vi "Polynomial Eigenvalue Problem (DBL, Spec Case).vi"(10 "output option":i32(ring)=1 items=["eigenvalues", "eigenvalues & vectors"], 11 "Input Matrices":dbl[][][](array[numeric])) -> (0 "error":i32, 2 "Eigenvectors":T1, 3 "Eigenvalues":cdb[](array[numeric]))   [LabVIEW 2020, in "NI_AALPro.lvlib"]
uses:
  <vilib>/Analysis/NI_AALPro.lvlib
  <vilib>/Analysis/Matrix/Datatypes/ComplexMatrix.ctl
  <vilib>/Analysis/7linalg.llb/Real Generalized Eigenvalues and Vectors.vi
  <vilib>/Analysis/7linalg.llb/Real Eigenvalues and Vectors.vi
  <vilib>/Analysis/Matrix/NI_Matrix.lvlib
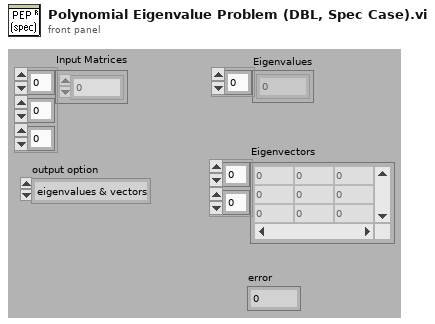
[diagram p1: front panel]
types:
  T1 = typedef "NI_Matrix.lvlib/ComplexMatrix.ctl" = cdb[][]
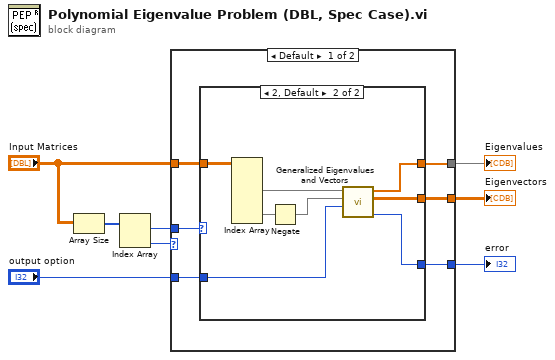
[diagram p0: block diagram]
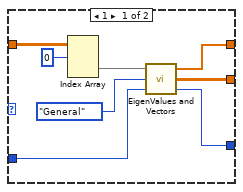
[diagram p2: hidden frame]
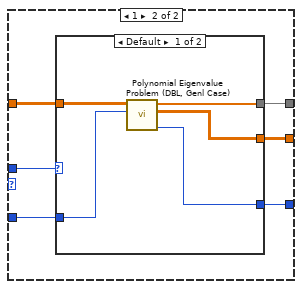
[diagram p3: hidden frame]
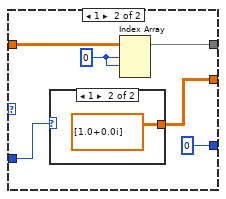
[diagram p4: hidden frame]
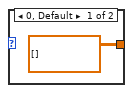
[diagram p5: hidden frame]
diagram:
  n1 = Array Size(array="Input Matrices") -> (size(s)=w8:i32[])
  n2 = Index Array(array=w8) -> (element #1=w6:i32, element #2=w7:i32)  [unwired: 2 in]
  n3 = case shown="Default" w7 {
    tunnel: w6 -> [w14 w36]
    tunnel: "Input Matrices" -> [w13 w35]
    tunnel: [w12 w34] -> w4
    tunnel: [w11 w33] -> w3
    tunnel: [w10 w32] -> w2
    tunnel: "output option" -> [w9 w31]
    frame Default {
      n4 = case shown="2, Default" w14 {
        tunnel: w13 -> [w22 w30]
        tunnel: [w18 w26] -> w12
        tunnel: [w17 w25] -> w11
        tunnel: [w16 w24] -> w10
        tunnel: w9 -> [w15 w23]
        frame 1 {
          n5 = Index Array(array=w22, index (dim 0)=0 ("index (page)")) -> (element=w20:dbl[][])  [unwired: 2 in]
          n6 = call-poly <vilib>:"EigenValues and Vectors.vi"("output option"=w15, "matrix type"=enum32{"General", "Symmetric"}."General", "Input Matrix"=w20) -> ("error"=w16:i32, "Eigenvectors"=w17:T1, "Eigenvalues"=w18:cdb[])
        }
        frame 2, Default {
          n7 = Index Array(array=w30) -> (element #1=w28:dbl[][], element #2=w29:dbl[][])  [unwired: 6 in]
          n8 = Negate(x=w29) -> (-x=w27:dbl[][])
          n9 = call-poly <vilib>:"Generalized Eigenvalues and Vectors.vi"("output option"=w23, "B"=w27, "A"=w28) -> ("error"=w24:i32, "Eigenvectors"=w25:T1, "Eigenvalues"=w26:cdb[])  [unwired: 3 in]
        }
      }
    }
    frame 1 {
      n10 = case shown="Default" w36 {
        tunnel: w35 -> [w41 w46]
        tunnel: [w40 w44] -> w34
        tunnel: [w39 w42] -> w33
        tunnel: [w38 0 ("error")] -> w32
        tunnel: w31 -> [w37 w43]
        frame Default {
          n11 = call <vilib>:"Polynomial Eigenvalue Problem (DBL, Genl Case).vi"("output option"=w37, "Input Matrices"=w41) -> ("error"=w38:i32, "Eigenvectors"=w39:T1, "Eigenvalues"=w40:cdb[])  [unwired: 7 in]
        }
        frame 1 {
          w45 = 0 ("index (page)")
          n12 = case shown="1" w43 {
            tunnel: [T1 [] ("Eigenvectors") T1 [[1.0+0.0i]] ("Eigenvectors")] -> w42
            frame 0, Default {
            }
            frame 1 {
            }
          }
          n13 = Index Array(array=w46, index (dim 0)=w45, index (dim 1)=w45) -> (element=w44:dbl[])  [unwired: 1 in]
        }
      }
    }
  }
  "Eigenvalues" <- w4
  "Eigenvectors" <- w3
  "error" <- w2
